vi "英维克设定参数对话框.vi"() -> (1 "参数 2":u16=3000, 2 "设定参数（定点数）选择 2":T1(ring), 3 "确定?":bool)   [LabVIEW 2016, in "环境动力监测库.lvlib" / "空调库.lvlib"]
panel:
  in  "参数":u16=3000
  in  "设定参数（定点数）选择":T1(ring)
  in  "取消":bool
  in  "确定":bool
  # "设定参数选择"
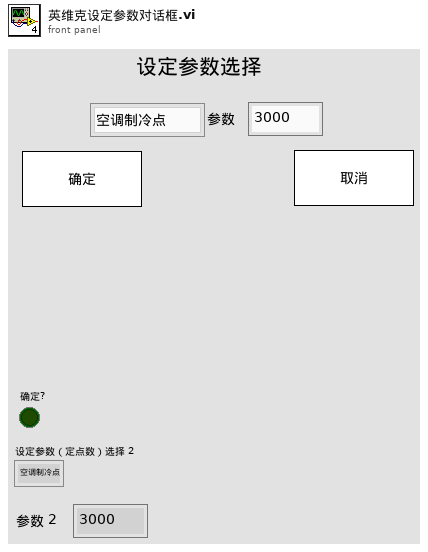
[diagram p1: front panel]
types:
  T1 = enum16{"空调制冷点", "空调制冷回差", "加热点", "加热回差", "高温点", "低温点", "高湿点", "内风机停止点"}
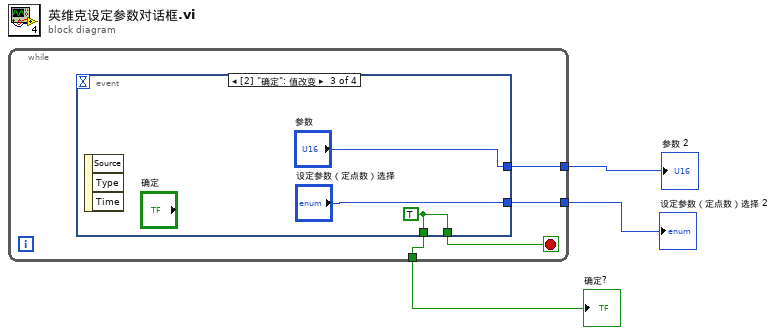
[diagram p0: block diagram]
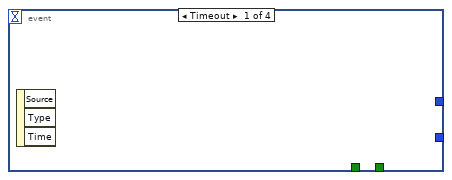
[diagram p2: hidden frame]
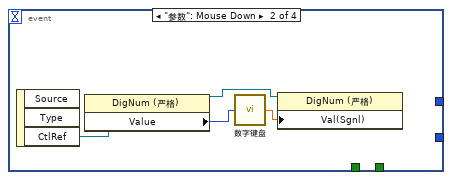
[diagram p3: hidden frame]
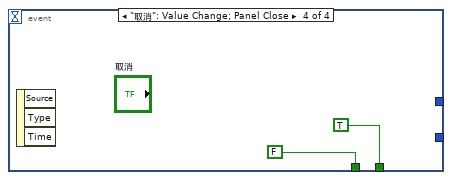
[diagram p4: hidden frame]
diagram:
  n1 = while {
    tunnel: [w7] -> w2
    tunnel: [w5] -> w3
    tunnel: [w4] -> w1
    stop <- w6 stop-if-true
    n2 = event shown="[2] \"确定\": 值改变" {
      selector: _ -> [_ _ _ _]
      dyn-events: _ -> [_ _ _ _]
      timeout: _ -> [_ _ _ _]
      tunnel: [_ _ w14 TRUE] -> w6
      tunnel: [_ _ "参数" _] -> w7
      tunnel: [_ _ w14 FALSE] -> w5
      tunnel: [_ _ "设定参数（定点数）选择" _] -> w4
      event Timeout {
        n3 = event-data() -> ()  [unwired: 1 in, 3 out]
      }
      event "参数": Mouse Down {
        n4 = event-data() -> ("CtlRef"=w11:refnum<vi>)  [unwired: 1 in, 2 out]
        n5 = property class="DigNum (严格)"(reference=w11) -> (reference out=w8:refnum<vi>, "Value"=w10:u16)  [unwired: 1 in, 1 out]
        n6 = call "数字键盘.vi"("OldNumber"=w10) -> ("NewNumber"=w9:sgl)
        n7 = property class="DigNum (严格)"(reference=w8, "Val(Sgnl)"=w9) -> ()  [unwired: 1 in, 2 out]
      }
      event "确定": Value Change {
        w14 = TRUE
        n8 = event-data() -> ()  [unwired: 1 in, 3 out]
      }
      event "取消": Value Change; Panel Close {
        n9 = event-data() -> ()  [unwired: 1 in, 3 out]
      }
    }
  }
  "确定?" <- w3
  "参数 2" <- w2
  "设定参数（定点数）选择 2" <- w1
